vi "update_expSD.vi"(0 "Experiment in":refnum<class "Experiment.lvclass">, 1 "Experiments groups in":refnum<class "Experiments_group.lvclass">[](array[class]), 2 "group":u16, 3 "error in (no error)":errorcluster, 4 "exp selected":i32) -> (5 "Experiments groups out":refnum<class "Experiments_group.lvclass">[](array[class]), 6 "error out":errorcluster)   [LabVIEW 2015]
uses:
  Classes/Experiments_group.lvclass
  Classes/Experiment.lvclass
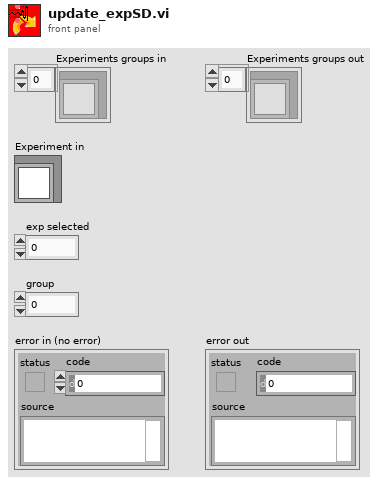
[diagram p1: front panel]
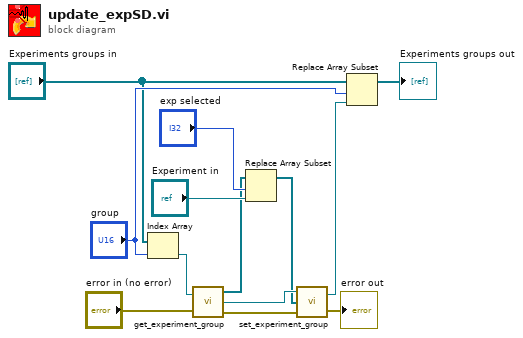
[diagram p0: block diagram]
diagram:
  n1 = Index Array(array="Experiments groups in", index="group") -> (element=w1:refnum<class "Experiments_group.lvclass">)
  n2 = call-dynamic "get_experiment_group.vi"("Experiments_group.lvclass in"=w1, "error in (no error)"="error in (no error)") -> ("Experiments"=w2:refnum<class "Experiment.lvclass">[], "Experiments_group.lvclass out"=w6:refnum<class "Experiments_group.lvclass">, "error out"=w12:errorcluster)
  n3 = Replace Array Subset(array=w2, new element="Experiment in", index="exp selected") -> (w5:refnum<class "Experiment.lvclass">[])
  n4 = call-dynamic "set_experiment_group.vi"("error in (no error)"=w12, "Experiments"=w5, "Experiments_group.lvclass in"=w6) -> ("error out"=→"error out":errorcluster, "Experiments_group.lvclass out"=w9:refnum<class "Experiments_group.lvclass">)
  n5 = Replace Array Subset(array="Experiments groups in", new element=w9, index="group") -> (→"Experiments groups out":refnum<class "Experiments_group.lvclass">[])
